vi "Image to base64.vi"(8 "error in (no error)":errorcluster, 10 "string in (not encoded)":string) -> (0 "error out":errorcluster, 2 "string out (base64-encoded)":string)   [LabVIEW 2019]
uses:
  <vilib>/picture/picture.llb/imagedata.ctl
panel:
  out "image data":T1
  in  "unsigned byte array":u8[](array[numeric])
  # "Overview: This example demonstrates how to encode to Base64.\nRequirements: LabVIEW Base Development System 2012 (or compatible)\nInstructions:\n1. Enter a string\n2. Run the VI"
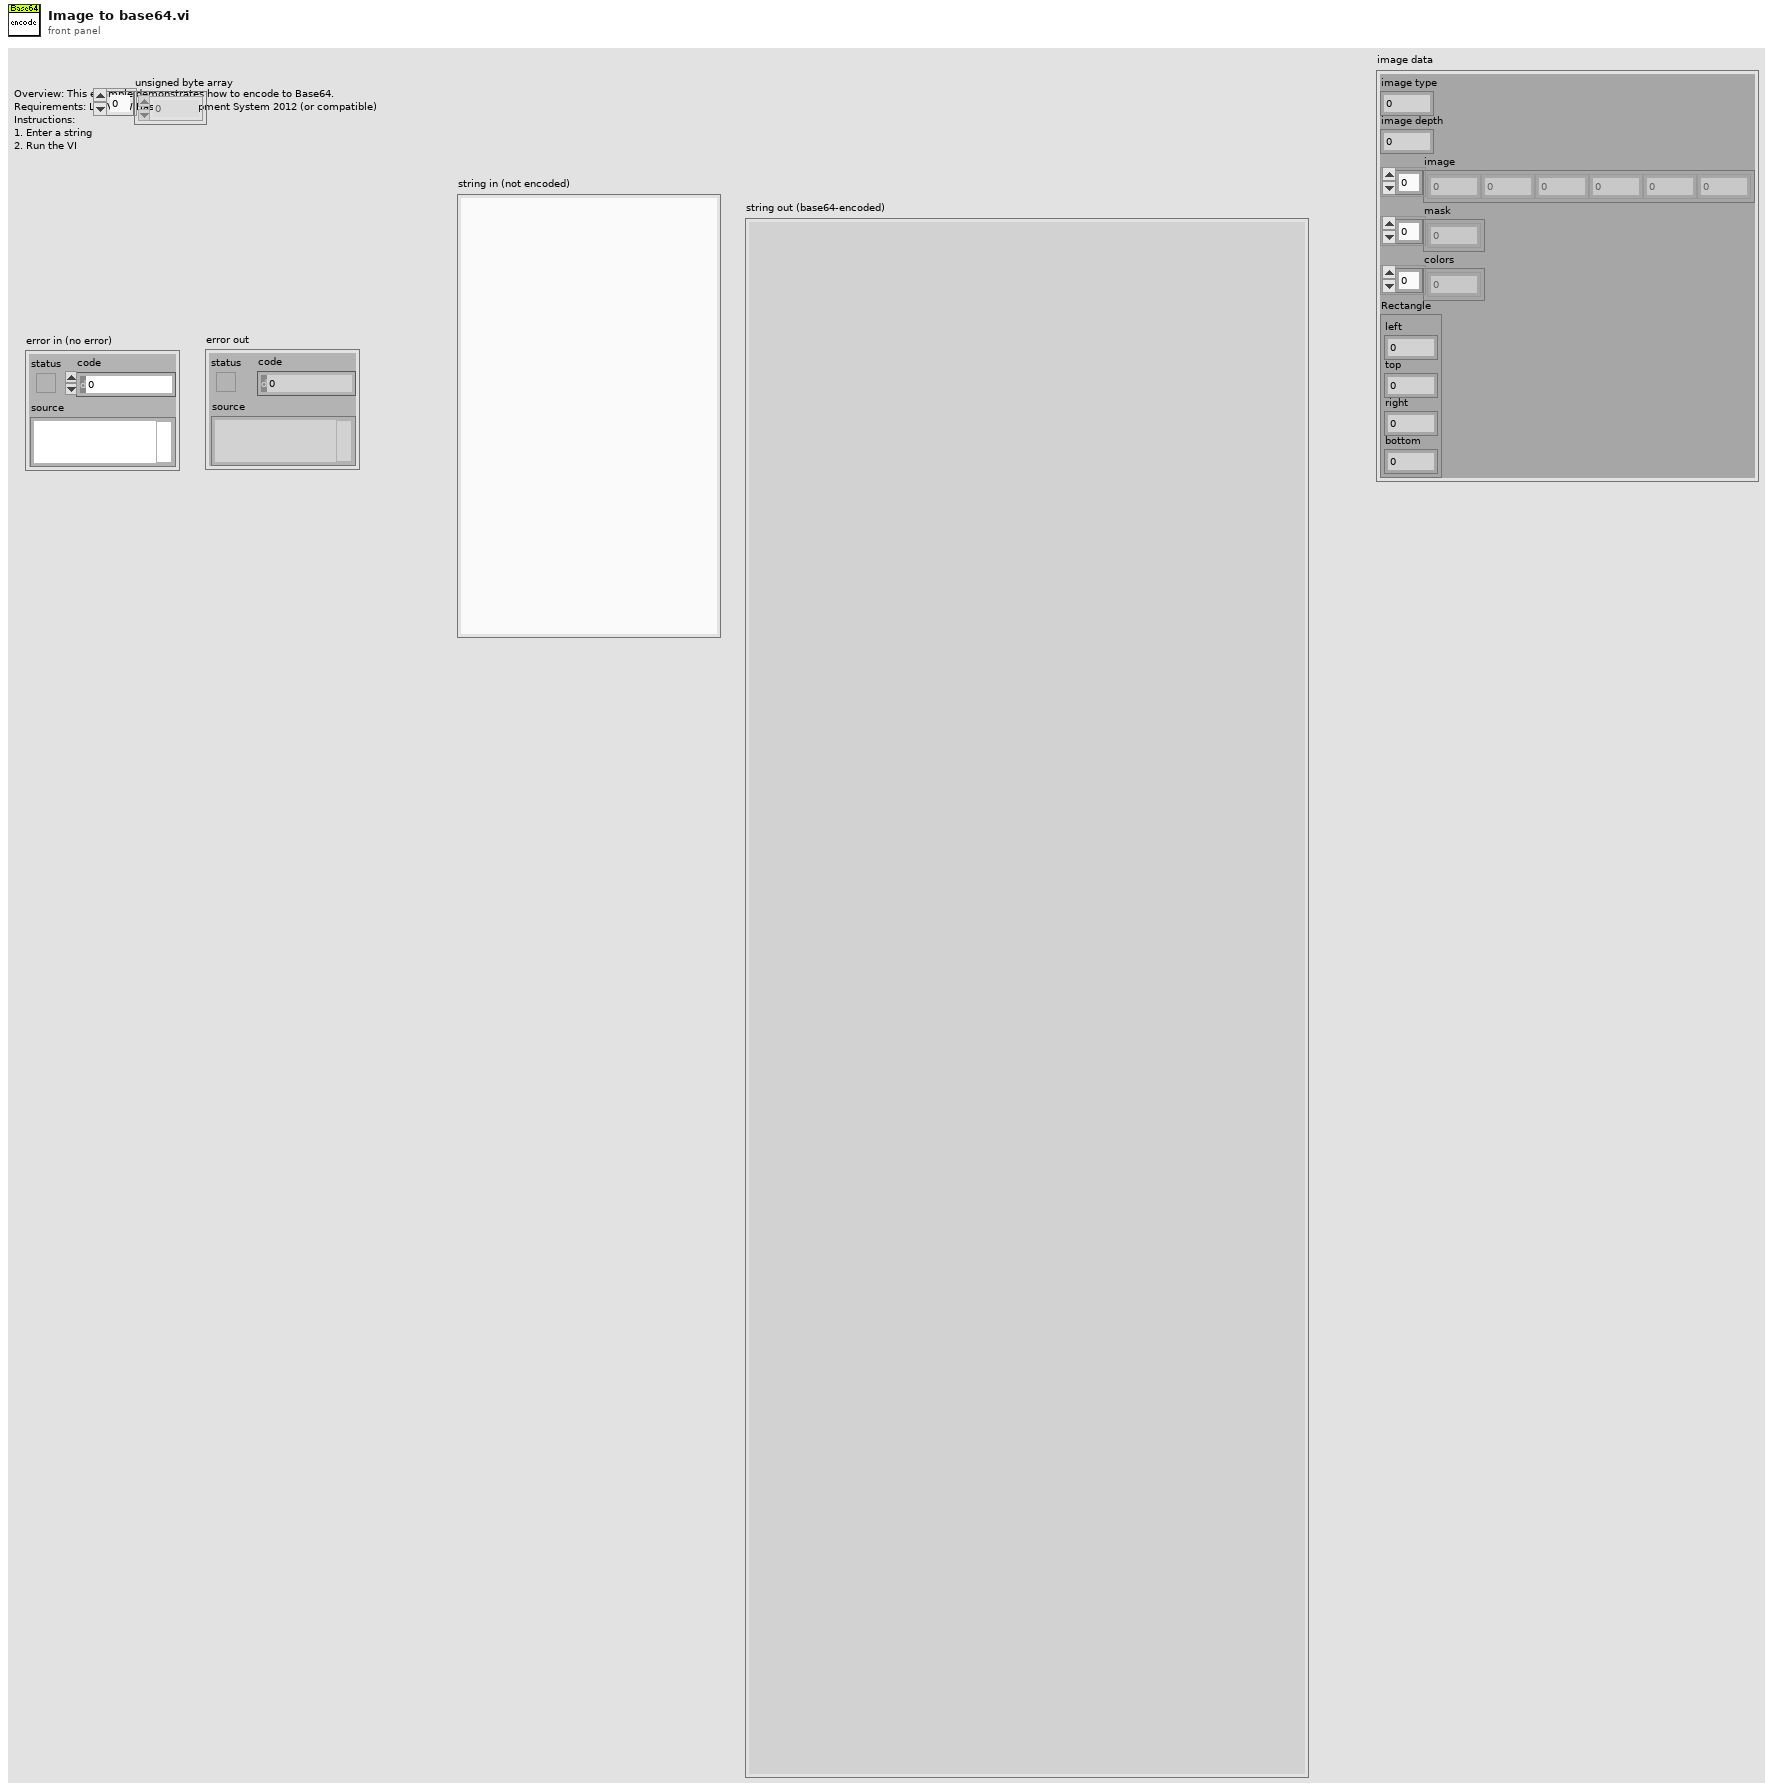
[diagram p1: front panel]
types:
  T1 = typedef "imagedata.ctl" = cluster{"image type":i32, "image depth":i32, "image":u8[], "mask":u8[], "colors":u32[], "Rectangle":cluster{"left":i16, "top":i16, "right":i16, "bottom":i16}}
  T2 = cluster{"image[0]":u8, "image[1]":u8, "image[2]":u8}
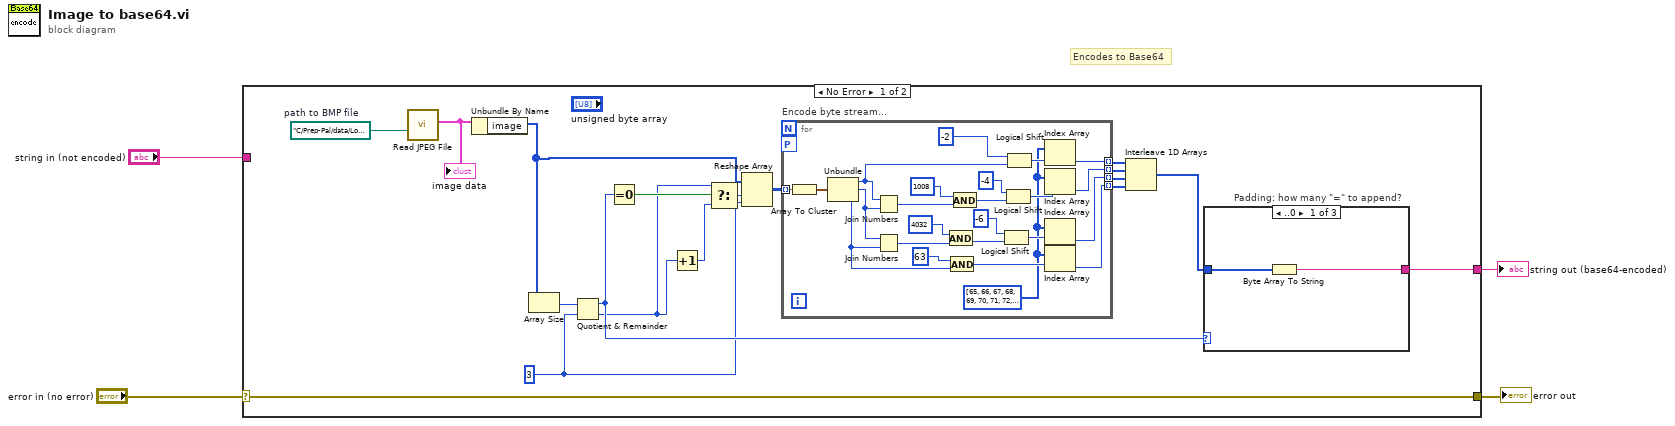
[diagram p0: block diagram]
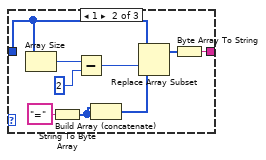
[diagram p2: hidden frame]
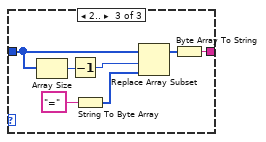
[diagram p3: hidden frame]
diagram:
  # "Encodes to Base64"
  n1 = case shown="No Error" "error in (no error)" {
    selector: "error in (no error)" -> [w22 w66]
    tunnel: "string in (not encoded)" -> [_ w65]
    tunnel: [w22 w66] -> w2
    tunnel: [w8 w65] -> w1
    frame No Error {
      w7 = path "C:/Prep-Pal/data/Logo.jpg"  # path to BMP file
      w11 = 3 ("y")
      n2 = call <vilib>:"Read JPEG File.vi"("path to JPEG file"=w7) -> ("image data"=w6:T1)  [unwired: 8 in, 2 out]
      "image data" <- w6
      n3 = Unbundle By Name(w6) -> ("image"=w5:u8[])
      n4 = Array Size(array=w5) -> (size(s)=w19:i32)
      n5 = Quotient & Remainder(x=w19, y=w11) -> (x-y*floor(x/y)=w20:i32, floor(x/y)=w13:i32)
      n6 = Equal To 0?(x=w20) -> (x = 0?=w21:bool)
      n7 = Increment(x=w13) -> (x+1=w14:i32)
      n8 = Select(t=w13, s=w21, f=w14) -> (s? t:f=w10:i32)
      n9 = Reshape Array(w5, w10, w11) -> (w9:u8[][])
      n10 = for "Encode byte stream..." {
        tunnel: [w25] -> w15 mode=indexing
        tunnel: [w26] -> w16 mode=indexing
        tunnel: [w27] -> w17 mode=indexing
        tunnel: [w28] -> w18 mode=indexing
        workers-P: _ -> [_]
        tunnel: w9 -> [w23] mode=indexing
        w24 = u8[] [65, 66, 67, 68, 69, 70, 71, 72, 73, 74, 75, 76, 77, 78, 79, 80, 81, 82, 83, 84, 85, 86, 87, 88, 89, 90, 97, 98, 99, 100, 101, 102, 103, 104, 105, 106, 107, 108, 109, 110, 111, 112, 113, 114, 115, 116, 117, 118, 119, 120, 121, 122, 48, 49, 50, 51, 52, 53, 54, 55, 56, 57, 43, 47] ("unsigned byte array")
        n11 = Array To Cluster(array=w23) -> (cluster=w46:T2)
        n12 = Unbundle(w46) -> ("image[0]"=w35:u8, "image[1]"=w40:u8, "image[2]"=w34:u8)
        n13 = Join Numbers(hi=w35, lo=w40) -> ((hi.lo)=w44:u16)
        n14 = Join Numbers(hi=w40, lo=w34) -> ((hi.lo)=w39:u16)
        n15 = And(x=u16 4032, y=w39) -> (x .and. y?=w37:u16)
        n16 = And(x=u8 63, y=w34) -> (x .and. y?=w29:u8)
        n17 = And(x=u16 1008, y=w44) -> (x .and. y?=w42:u16)
        n18 = Logical Shift(y=i8 -6, x=w37) -> (x << y=w30:u16)
        n19 = Logical Shift(y=i8 -4, x=w42) -> (x << y=w31:u16)
        n20 = Logical Shift(y=i8 -2, x=w35) -> (x << y=w32:u8)
        n21 = Index Array(array=w24, index=w32) -> (element=w28:u8)
        n22 = Index Array(array=w24, index=w31) -> (element=w27:u8)
        n23 = Index Array(array=w24, index=w30) -> (element=w26:u8)
        n24 = Index Array(array=w24, index=w29) -> (element=w25:u8)
      }
      n25 = Interleave 1D Arrays(w18, w17, w16, w15) -> (w12:u8[])
      n26 = case "Padding: how many \"=\" to append?" shown="..0" w20 {
        tunnel: [w47 w54 w63] -> w8
        tunnel: w12 -> [w48 w52 w62]
        frame ..0 {
          n27 = Byte Array To String(unsigned byte array=w48) -> (string=w47:string)
        }
        frame 1 {
          n28 = Array Size(array=w52) -> (size(s)=w53:i32)
          n29 = String To Byte Array(string="=") -> (unsigned byte array=w50:u8[])
          n30 = Subtract(x=w53, y=2) -> (x-y=w56:i32)
          n31 = Build Array (concatenate)(w50, w50) -> (w49:u8[])
          n32 = Replace Array Subset(array=w52, new element=w49, index=w56) -> (w55:u8[])
          n33 = Byte Array To String(unsigned byte array=w55) -> (string=w54:string)
        }
        frame 2.. {
          n34 = Array Size(array=w62) -> (size(s)=w58:i32)
          n35 = Decrement(x=w58) -> (x-1=w59:i32)
          n36 = String To Byte Array(string="=") -> (unsigned byte array=w60:u8[])
          n37 = Replace Array Subset(array=w62, new element=w60, index=w59) -> (w64:u8[])
          n38 = Byte Array To String(unsigned byte array=w64) -> (string=w63:string)
        }
      }
    }
    frame Error {
    }
  }
  "string out (base64-encoded)" <- w1
  "error out" <- w2
